vi "EOL Analog Data Acquisition v1.1.vi"(7 "ms":refnum<vi>, 8 "error in":errorcluster, 9 "Base Path":path=path "C:/Labview Code", 11 "Exit Refnum":refnum<vi>) -> (0 "error out":errorcluster)   [LabVIEW 2018]
uses:
  <vilib>/DAQmx/read.llb/DAQmx Read (Analog 2D DBL NChan NSamp).vi
  <vilib>/DAQmx/configure/timing.llb/DAQmx Timing (Sample Clock).vi
  <vilib>/DAQmx/miscellaneous.llb/DAQmx Fill In Error Info.vi
panel:
  out "error out":errorcluster
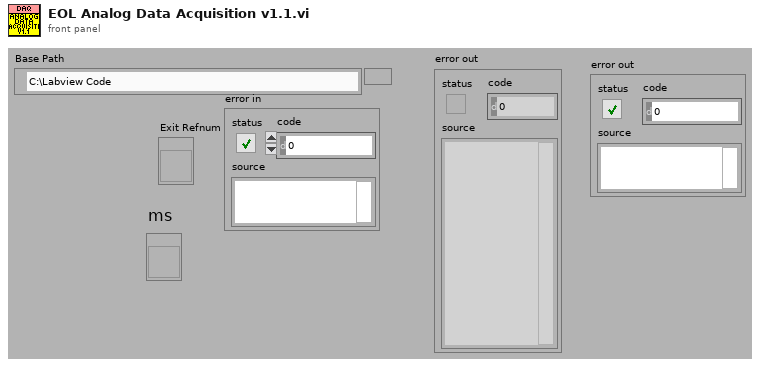
[diagram p1: front panel]
types:
  T1 = cluster{"AI Task ID":refnum<k21>, "Hall State In Array":i32[], "Remaining Data Array":cluster{"Hall and Current Data":sgl[][]}[], "No. of BMW Motors":i32, "Base Path":path, "error in":errorcluster}
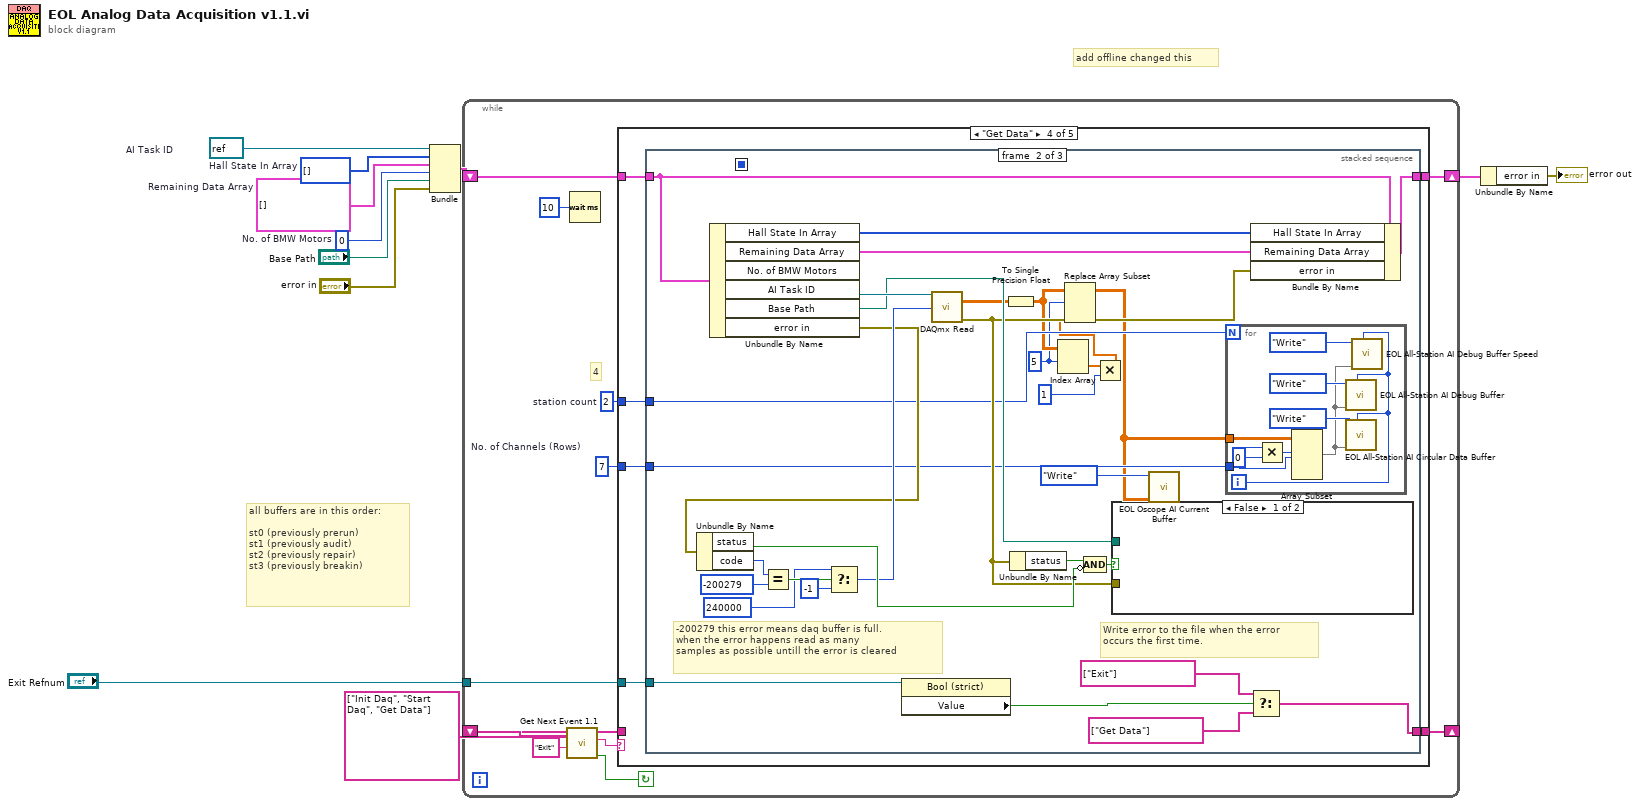
[diagram p0: block diagram]
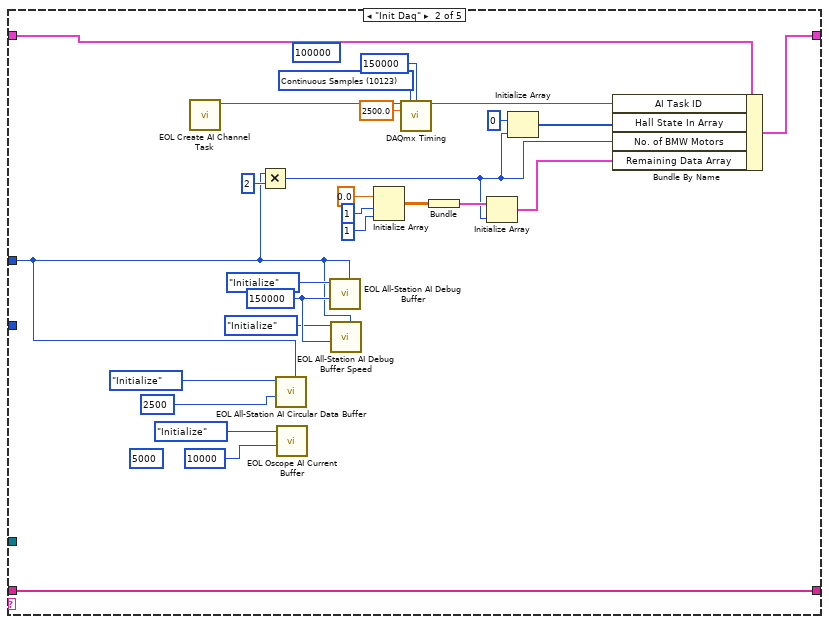
[diagram p3: hidden frame]
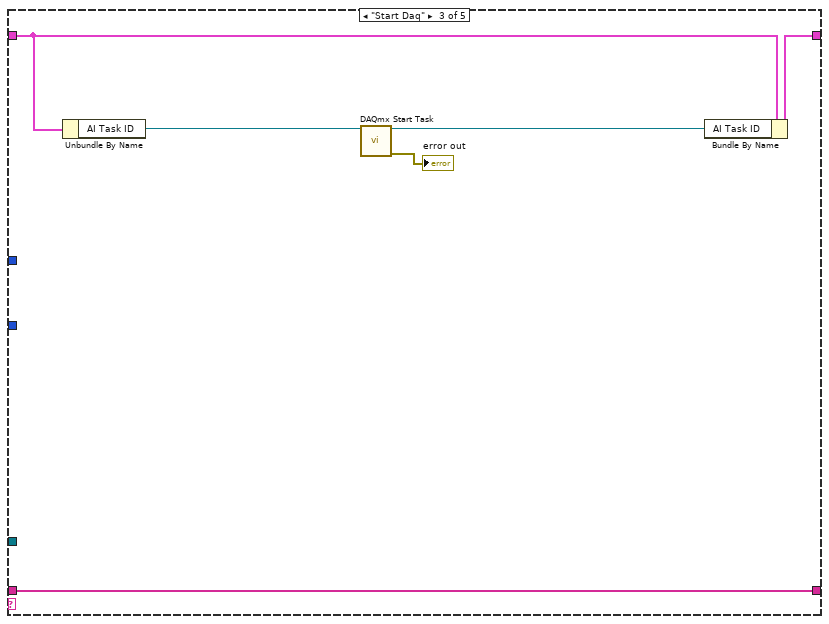
[diagram p4: hidden frame]
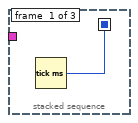
[diagram p5: hidden frame]
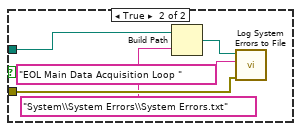
[diagram p6: hidden frame]
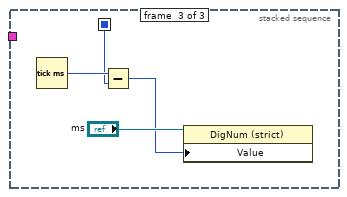
[diagram p7: hidden frame]
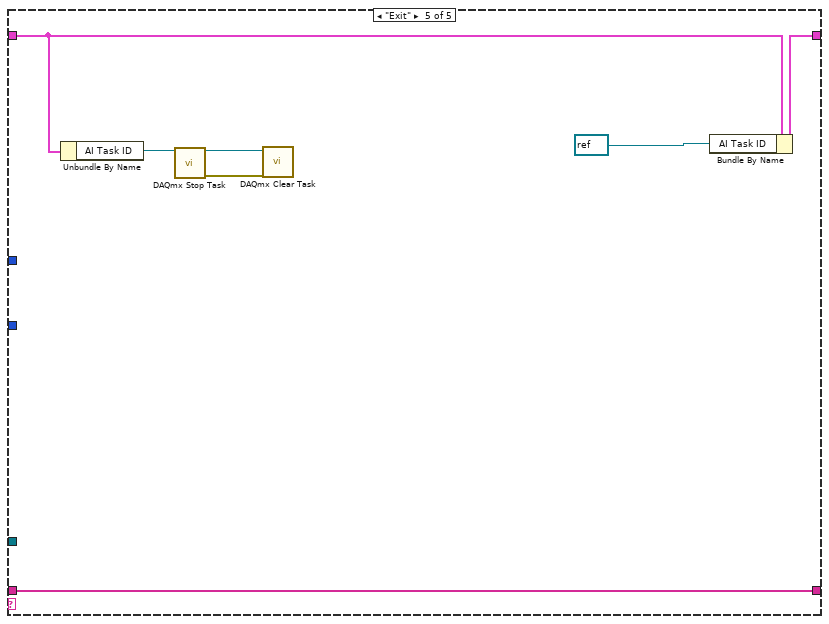
[diagram p8: hidden frame]
diagram:
  w5 = 0  # No. of BMW Motors
  w10 = cluster{"Hall and Current Data":sgl[][]}[] []  # Remaining Data Array
  w9 = i32[] []  # Hall State In Array
  w7 = refnum<k21> refnum  # AI Task ID
  # "add offline changed this"
  # "all buffers are in this order:\n\nst0 (previously prerun)\nst1 (previously audit)\nst2 (previously repair)\nst3 (previously breakin)"
  n1 = Bundle("AI Task ID"=w7, "Hall State In Array"=w9, "Remaining Data Array"=w10, "No. of BMW Motors"=w5, "Base Path"="Base Path", "error in"="error in") -> (w8:T1)  [unwired: 1 in]
  n2 = while {
    shift-right: [w20] -> _
    shift-left: string[] ["Init Daq", "Start Daq", "Get Data"] ("event queue out") -> [w19]
    shift-right: [w17] -> w2
    shift-left: w8 -> [w18]
    tunnel: "Exit Refnum" -> [w14]
    stop <- w15 continue-if-true
    w12 = 2  # station count
    w13 = 7  # No. of Channels (Rows)
    # "4"
    n3 = call "Get Next Event 1.1.vi"("Exit Event"="Exit", "event queue in"=w19) -> ("Condition (Exit:F)"=w15:bool, "next event"=w22:string, "event queue out"=w21:string[])  [unwired: 6 in, 1 out]
    n4 = Wait (ms)(milliseconds to wait=u32 10) -> ()  [unwired: 1 out]
    n5 = case shown="\"Get Data\"" w22 {
      tunnel: w21 -> [w25 w51 w57 _ w121]
      tunnel: [w25 w51 w57 w63 w121] -> w20
      tunnel: w18 -> [w24 w31 w54 w61 w116]
      tunnel: [w24 w40 w55 w60 w117] -> w17
      tunnel: w14 -> [_ _ _ w62 _]
      tunnel: w13 -> [_ _ _ w59 _]
      tunnel: w12 -> [_ w27 _ w58 _]
      frame "Error", Default {
      }
      frame "Init Daq" {
        (unwired) 100000 ("samples per channel")
        (unwired) 5000 ("Buffer Size (No. of Columns)")
        w29 = 150000 ("Buffer Size (seconds/2500)")
        w50 = 10123 items=["Finite Samples"=10178, "Continuous Samples"=10123, "Hardware Timed Single Point"=12522] ("sample mode")
        n6 = call "EOL Create AI Channel Task.vi"() -> ("Analog Input Task"=w26:refnum<k21>)  [unwired: 10 in, 1 out]
        n7 = Multiply(x=w27, y=2) -> (x*y=w35:i32)
        n8 = call "EOL All-Station AI Circular Data Buffer.vi"("number of stations"=w27, "Buffer Size (seconds/2500)"=2500 ("Buffer Size (No. of Columns)"), "Mode"=enum16{"Initialize", "Read", "Write"}."Initialize") -> ()  [unwired: 8 in, 1 out]
        n9 = call "EOL Oscope AI Current Buffer.vi"("Buffer Size (seconds/2500)"=10000 ("Buffer Size (No. of Columns)"), "Mode"=enum16{"Initialize", "Read", "Write"}."Initialize") -> ()  [unwired: 9 in, 1 out]
        n10 = call "EOL All-Station AI Debug Buffer.vi"("number of stations"=w27, "Buffer Size (seconds/2500)"=w29, "Mode"=enum16{"Initialize", "Read", "Write"}."Initialize") -> ()  [unwired: 8 in, 1 out]
        n11 = call "EOL All-Station AI Debug Buffer Speed.vi"("number of stations"=w27, "Buffer Size (seconds/2500)"=w29, "Mode"=enum16{"Initialize", "Read", "Write"}."Initialize") -> ()  [unwired: 8 in, 1 out]
        n12 = Initialize Array(sgl 0.0 ("Last Hall State In"), 1 ("dimension size"), 1 ("dimension size")) -> (w42:sgl[][])
        n13 = call-poly <vilib>:"DAQmx Timing.vi"("task/channels in"=w26, "sample mode"=w50, "samples per channel"=150000, "rate"=2500.0) -> ("task out"=w37:refnum<k21>)  [unwired: 10 in, 1 out]
        n14 = Bundle(w42) -> (w41:cluster{sgl[][]})  [unwired: 1 in]
        n15 = Initialize Array(w41, w35) -> (w39:cluster{sgl[][]}[])
        n16 = Initialize Array(0 ("Last Hall State In"), w35) -> (w38:i32[])
        n17 = Bundle By Name(cluster=w31, "AI Task ID"=w37, "Hall State In Array"=w38, "No. of BMW Motors"=w35, "Remaining Data Array"=w39) -> (w40:T1)
      }
      frame "Start Daq" {
        n18 = Unbundle By Name(w54) -> ("AI Task ID"=w52:refnum<k21>)
        n19 = call <vilib>:"DAQmx Start Task.vi"("task/channels in"=w52) -> ("task out"=w56:refnum<k21>, "error out"=→"error out":errorcluster)  [unwired: 13 in]
        n20 = Bundle By Name(cluster=w54, "AI Task ID"=w56) -> (w55:T1)
      }
      frame "Get Data" {
        n21 = stacked-sequence {
          seq-local: [w64 _ _] -> [_ _ w113]
          tunnel: [_ w94 _] -> w63
          tunnel: w62 -> [_ w91 _]
          tunnel: w61 -> [_ w90 _]
          tunnel: [_ w89 _] -> w60
          tunnel: w59 -> [_ w74 _]
          tunnel: w58 -> [_ w73 _]
          frame #0 {
            n22 = Tick Count (ms)() -> (millisecond timer value=w64:u32)
          }
          frame #1 {
            w67 = 5 ("禁用的索引 (列)")
            # "Write error to the file when the error\noccurs the first time."
            # "-200279 this error means daq buffer is full.\nwhen the error happens read as many \nsamples as possible untill the error is cleared"
            n23 = Unbundle By Name(w90) -> ("Hall State In Array"=w66:i32[], "Remaining Data Array"=w65:cluster{"Hall and Current Data":sgl[][]}[], "AI Task ID"=w92:refnum<k21>, "Base Path"=w79:path, "error in"=w78:errorcluster)  [unwired: 1 out]
            n24 = Unbundle By Name(w78) -> ("status"=w81:bool, "code"=w84:i32)
            n25 = Equal?(x=w84, y=-200279 ("code 2")) -> (x = y?=w88:bool)
            n26 = Select(t=240000 ("number of samples per channel"), s=w88, f=-1) -> (s? t:f=w80:i32)
            n27 = property on="Property Node" class="Bool (strict)"(reference=w91) -> ("Value"=w93:bool)  [unwired: 1 in, 2 out]
            n28 = call-poly <vilib>:"DAQmx Read.vi"("task/channels in"=w92, "number of samples per channel"=w80) -> ("data"=w75:dbl[][], "error out"=w77:errorcluster)  [unwired: 11 in, 1 out]
            n29 = To Single Precision Float(number=w75) -> (single precision float=w72:sgl[][])
            n30 = Unbundle By Name(w77) -> ("status"=w83:bool)
            n31 = Index Array(array=w72, index (row)=w67) -> (element=w70:sgl[])  [unwired: 1 in]
            n32 = Compound Arithmetic op=AND(w83, invert w81) -> (w82:bool)
            n33 = Multiply(x=w70, y=1) -> (x*y=w68:sgl[])
            n34 = Replace Array Subset(array=w72, new element=w68, index (row)=w67) -> (w71:sgl[][])  [unwired: 1 in]
            n35 = case shown="False" w82 {
              tunnel: w77 -> [_ w109]
              tunnel: w79 -> [_ w108]
              frame False {
              }
              frame True {
                n36 = Build Path(base path=w108, name or relative path="System\\System Errors\\System Errors.txt") -> (appended path=w107:path)
                n37 = call "Log System Errors to File.vi"("error out"=w109, "Comments"="EOL Main Data Acquisition Loop ", "Path"=w107) -> ()  [unwired: 9 out]
              }
            }
            n38 = call "EOL Oscope AI Current Buffer.vi"("Data to Write (Ch-Ro, Samp-Col)"=w71, "Mode"=enum16{"Initialize", "Read", "Write"}."Write") -> ()  [unwired: 9 in, 1 out]
            n39 = for {
              N: w73 -> [_]
              tunnel: w71 -> [w105]
              tunnel: w74 -> [w103]
              i -> [w99]
              n40 = Multiply(x=w103, y=0) -> (x*y=w104:i32)
              n41 = Array Subset(array=w105, index (row)=w104, length (row)=w103) -> (w98:sgl[][])  [unwired: 2 in]
              n42 = call "EOL All-Station AI Debug Buffer.vi"("station idx"=w99, "Data to Write (Ch-Ro, Samp-Col)"=w98, "Mode"=enum16{"Initialize", "Read", "Write"}."Write") -> ()  [unwired: 8 in, 1 out]
              n43 = call "EOL All-Station AI Circular Data Buffer.vi"("station idx"=w99, "Data to Write (Ch-Ro, Samp-Col)"=w98, "Mode"=enum16{"Initialize", "Read", "Write"}."Write") -> ()  [unwired: 8 in, 1 out]
              n44 = call "EOL All-Station AI Debug Buffer Speed.vi"("station idx"=w99, "Data to Write (Ch-Ro, Samp-Col)"=w98, "Mode"=enum16{"Initialize", "Read", "Write"}."Write") -> ()  [unwired: 8 in, 1 out]
            }
            n45 = Bundle By Name(cluster=w90, "Hall State In Array"=w66, "Remaining Data Array"=w65, "error in"=w77) -> (w89:T1)
            n46 = Select(t=string[] ["Exit"] ("event queue out"), s=w93, f=string[] ["Get Data"] ("event queue out")) -> (s? t:f=w94:string[])
          }
          frame #2 {
            n47 = Tick Count (ms)() -> (millisecond timer value=w114:u32)
            n48 = Subtract(x=w114, y=w113) -> (x-y=w111:u32)
            n49 = property class="DigNum (strict)"(reference="ms", "Value"=w111) -> ()  [unwired: 1 in, 2 out]
          }
        }
      }
      frame "Exit" {
        n50 = Unbundle By Name(w116) -> ("AI Task ID"=w115:refnum<k21>)
        n51 = call <vilib>:"DAQmx Stop Task.vi"("task/channels in"=w115) -> ("task out"=w120:refnum<k21>, "error out"=w119:errorcluster)  [unwired: 13 in]
        n52 = call <vilib>:"DAQmx Clear Task.vi"("task in"=w120, "error in"=w119) -> ()  [unwired: 13 in, 1 out]
        n53 = Bundle By Name(cluster=w116, "AI Task ID"=refnum<k21> refnum ("task out")) -> (w117:T1)
      }
    }
  }
  n54 = Unbundle By Name(w2) -> ("error in"=→"error out":errorcluster)
